vi "GUIQueueCreate.vi"(2 "error in (no error)":errorcluster) -> (0 "GUIError":errorcluster, 1 "GUIQueue":refnum<queue>)   [LabVIEW 2017]
uses:
  GUIQueueCluster.ctl
  GUIMessage.ctl
panel:
  in  "Queuename":string
  in  "GUIQueueCluster":T1={"GUIMessage"=enum."Channel1Value", "NumericValue"=0.0, "String"=""}
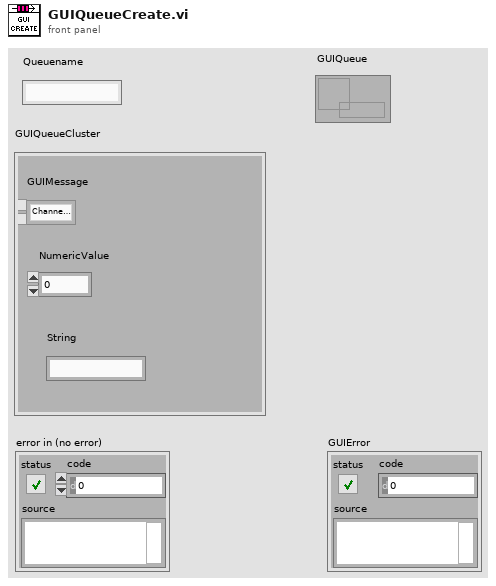
[diagram p1: front panel]
types:
  T1 = typedef "GUIQueueCluster.ctl" = cluster{"GUIMessage":T2, "NumericValue":dbl, "String":string}
  T2 = typedef "GUIMessage.ctl" = enum16{"StopSave", "Channel1Value", "Channel2Value", "Channel3Value", "ErrorSource", "CleanError", "StartChannel1", "StartChannel2", "StartChannel3", "StopChannel1", "StopChannel2", "StopChannel3", "Halt"}
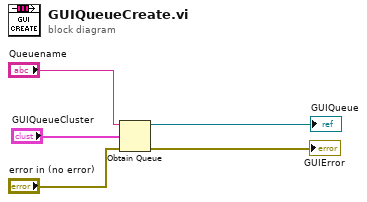
[diagram p0: block diagram]
diagram:
  n1 = Obtain Queue(name (unnamed)="Queuename", element data type="GUIQueueCluster", error in (no error)="error in (no error)") -> (queue out=→"GUIQueue":refnum<queue>, error out=→"GUIError":errorcluster)  [unwired: 2 in, 1 out]
